vi "Add Status Channel.vi"(8 "error in":errorcluster, 10 "name (empty = \"Status\")":string, 11 "message or subaddress":T1 format="%.0x") -> (0 "error out":errorcluster, 2 "status channel":T1 format="%.0x", 3 "message or subaddress out":T1 format="%.0x")   [LabVIEW 2020, in "AIM MIL-STD-1553 Scripting.lvlib"]
doc: "Adds a <b>status channel</b> to the specified <b>message or subaddress</b> section."
uses:
  AIM MIL-STD-1553 Scripting.lvlib
  <vilib>/NI VeriStand/Custom Device API/Custom Device Item Ref.ctl
  <vilib>/NI VeriStand/Custom Device API/Custom Device Channel.ctl
  <vilib>/NI VeriStand/Custom Device API/Custom Device Channel Type.ctl
  Constants.vi
  <vilib>/NI VeriStand/Custom Device API/Custom Device API.lvlib
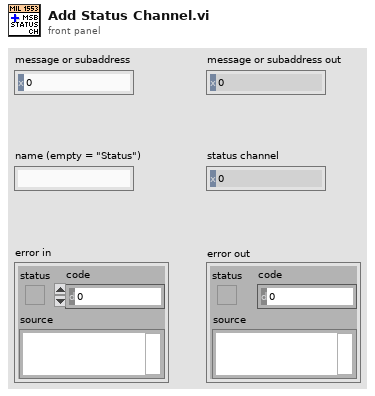
[diagram p1: front panel]
types:
  T1 = typedef "Custom Device API.lvlib/Custom Device Item Ref.ctl" = u64
  T2 = typedef "Custom Device API.lvlib/Custom Device Channel.ctl" = cluster{"Type":T3, "Units":string, "Default Value":dbl, "Faultable":bool, "Scalable":bool}
  T3 = typedef "Custom Device API.lvlib/Custom Device Channel Type.ctl" = enum16{"Input", "Output"}
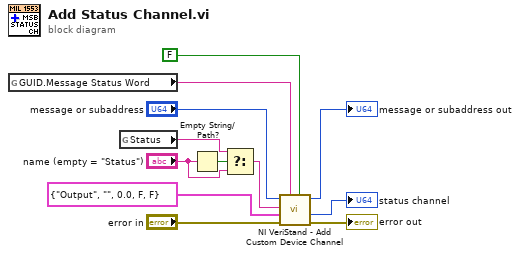
[diagram p0: block diagram]
diagram:
  n1 = global read "Constants.vi" "GUID.Message Status Word"() -> (w6:string)
  n2 = global read "Constants.vi" "Status"() -> (w5:string)
  n3 = Empty String/Path?(string/path="name (empty = \"Status\")") -> (empty?=w4:bool)
  n4 = Select(t=w5, s=w4, f="name (empty = \"Status\")") -> (s? t:f=w2:string)
  n5 = call <vilib>:"NI VeriStand - Add Custom Device Channel.vi"("Highlight? (F)"=FALSE, "GUID (Default Channel)"=w6, "error in (no error)"="error in", "Channel"=T2 {"Type"=enum."Output", "Units"="", "Default Value"=0.0, "Faultable"=FALSE, "Scalable"=FALSE}, "Channel Name"=w2, "Parent Ref in"="message or subaddress") -> ("error out"=→"error out":errorcluster, "Channel Ref"=→"status channel":T1, "Parent Ref out"=→"message or subaddress out":T1)  [unwired: 2 in, 1 out]
